vi "Read Image.vi"(0 "video in":refnum<class "MSC Video.lvclass">, 1 "image in":refnum<class "MSC Image.lvclass">, 5 "error in (no error)":errorcluster) -> (14 "video out":refnum<class "MSC Video.lvclass">, 15 "image out":refnum<class "MSC Image.lvclass">, 19 "error out":errorcluster)   [LabVIEW 2014, in "MSC Video.lvclass"]
doc: "Reads a frame from the camera and returns it as MSC Image.\nYou can use the image in connector to get around allocating and deallocation memory for each grabbed frame."
uses:
  MSC Video.lvclass
  MSC Image_class/MSC Image.lvclass
  MSC Video.lvclass/MSC Video.ctl
  Dependencies/x86/MSC I Process32.dll
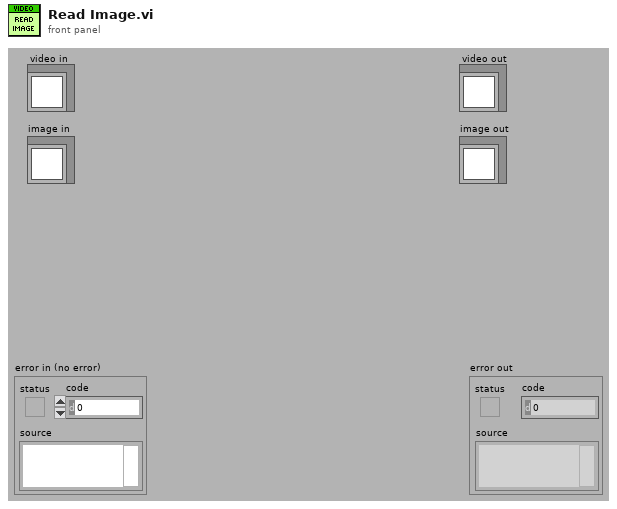
[diagram p1: front panel]
types:
  T1 = typedef "MSC Image.lvclass/Image.ctl" = cluster{"Pointer":u64, "Size":T2, "Image Type":T3, "Time Stamp":timestamp, "Variant":variant}
  T2 = typedef "MSC Image.lvclass/Size.ctl" = cluster{"Cols":i32, "Rows":i32}
  T3 = typedef "MSC Image.lvclass/Image Type.ctl" = i32
  T4 = typedef "MSC Video.lvclass/Video.ctl" = cluster{"Pointer":u64, "CamID":i32, "File Path":path, "Network Address":string, "opened":bool}
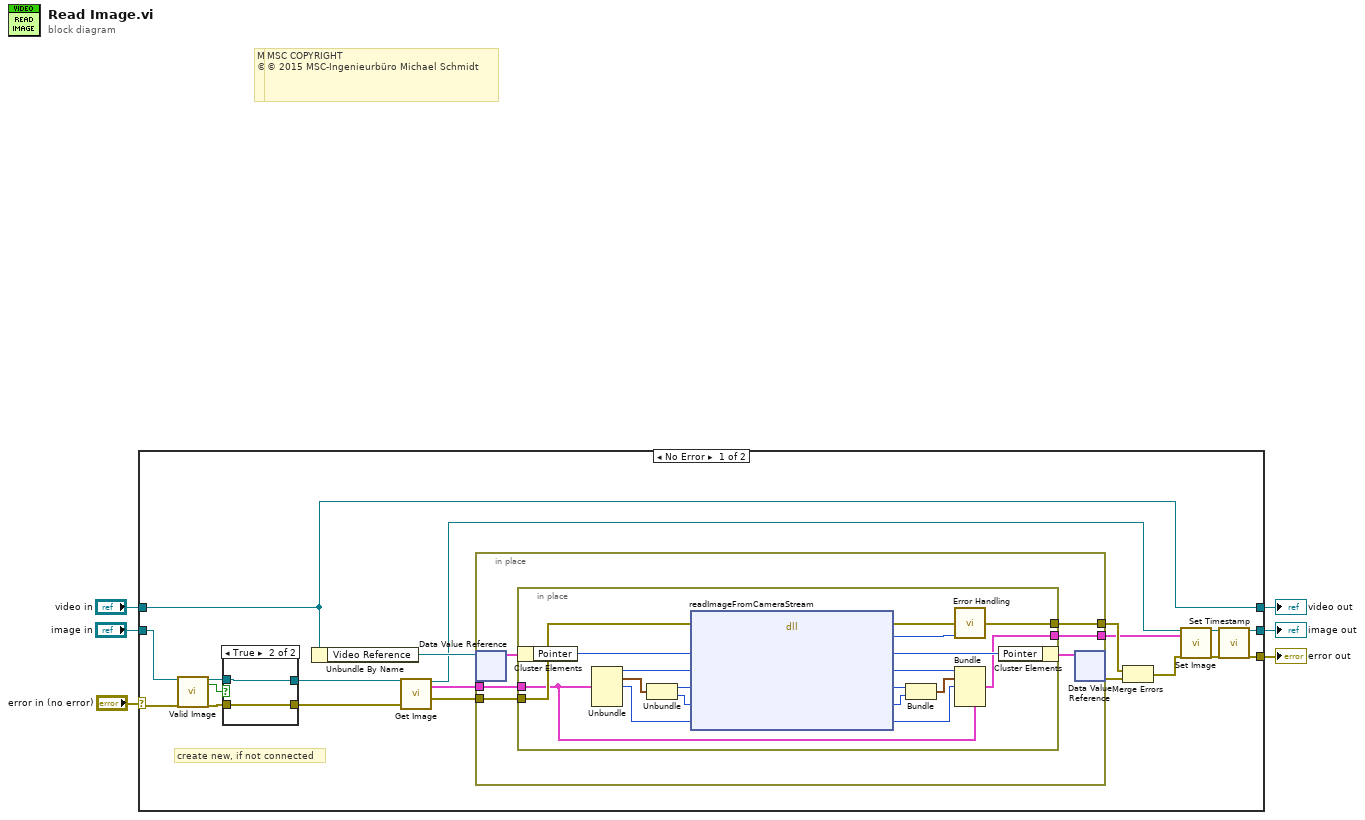
[diagram p0: block diagram]
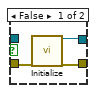
[diagram p2: hidden frame]
diagram:
  # "MSC COPYRIGHT\n© 2016 MSC-Ingenieurbüro Michael Schmidt"
  # "MSC COPYRIGHT\n© 2016 MSC-Ingenieurbüro Michael Schmidt"
  # "MSC COPYRIGHT\n© 2015 MSC-Ingenieurbüro Michael Schmidt"
  n1 = case shown="No Error" "error in (no error)" {
    selector: "error in (no error)" -> [w12 w58]
    tunnel: [w15 w58] -> w3
    tunnel: "video in" -> [w20 w57]
    tunnel: [w20 w57] -> w4
    tunnel: [w16 w56] -> w2
    tunnel: "image in" -> [w13 w56]
    frame No Error {
      # "create new, if not connected"
      n2 = call-dynamic "Valid Image.vi"("image in"=w13, "error in (no error)"=w12) -> ("image out"=w8:refnum<class "MSC Image.lvclass">, "Valid Image?"=w11:bool, "error out"=w9:errorcluster)  [unwired: 15 in]
      n3 = case shown="True" w11 {
        tunnel: [w28 w31] -> w10
        tunnel: w9 -> [w27 w31]
        tunnel: w8 -> [_ w30]
        tunnel: [w29 w30] -> w7
        frame False {
          n4 = call "Initialize.vi"("error in (no error)"=w27) -> ("image out"=w29:refnum<class "MSC Image.lvclass">, "error out"=w28:errorcluster)  [unwired: 17 in]
        }
        frame True {
        }
      }
      n5 = Unbundle By Name(w20) -> ("Video Reference"=w21:refnum<data-value>)
      n6 = call-dynamic "Get Image.vi"("image in"=w7, "error in (no error)"=w10) -> ("image out"=w18:refnum<class "MSC Image.lvclass">, "Image"=w24:T1, "error out"=w23:errorcluster)  [unwired: 15 in]
      n7 = in-place {
        in-place-border: w23 -> [w35]
        in-place-border: [w34] -> w25
        in-place-border: w24 -> [w33]
        in-place-border: [w32] -> w19
        n8 = in-place-dvr #1(w21) -> (w36:T4)  [unwired: 1 out]
        n9 = in-place {
          in-place-border: w35 -> [w39]
          in-place-border: [w42] -> w34
          in-place-border: w33 -> [w38]
          in-place-border: [w40] -> w32
          n10 = in-place-cluster #2(w36) -> ("Pointer"=w43:u64)
          n11 = Unbundle(w38) -> ("Pointer"=w44:u64, "Size"=w48:T2, "Image Type"=w47:T3)  [unwired: 2 out]
          n12 = Unbundle(w48) -> ("Cols"=w45:i32, "Rows"=w46:i32)
          n13 = dll-call lib="C:/Users/MSC/LabVIEW Projekte/LV 2014/MSC I-Process/user.lib/MSC-I Process/Dependencies/x86/MSC I Process*.dll" fn="readImageFromCameraStream"(error in=w39, "streamPointer"=w43, "pointer"=w44, "cols"=w45, "rows"=w46, "type"=w47) -> (error out=w54:errorcluster, "error"=w55:i32, "streamPointer"=w41:u64, "pointer"=w52:u64, "cols"=w50:i32, "rows"=w51:i32, "type"=w53:i32)  [unwired: 2 in, 1 out]
          n14 = Bundle("cols"=w50, "rows"=w51) -> (w49:cluster{"cols":i32, "rows":i32})  [unwired: 1 in]
          n15 = call "Error Handling.vi"("error in (no error)"=w54, "return type"=w55) -> ("error out"=w42:errorcluster)  [unwired: 12 in, 1 out]
          n16 = Bundle(cluster=w38, "Pointer"=w52, "Size"=w49, "Image Type"=w53) -> (w40:T1)  [unwired: 2 in]
          n17 = in-place-cluster #2("Pointer"=w41) -> (w37:T4)
        }
        n18 = in-place-dvr #1(w37) -> (w26:errorcluster)  [unwired: 1 out]
      }
      n19 = Merge Errors(w25, w26) -> (w22:errorcluster)
      n20 = call-dynamic "Set Image.vi"("image in"=w18, "Image"=w19, "error in (no error)"=w22) -> ("image out"=w17:refnum<class "MSC Image.lvclass">, "error out"=w14:errorcluster)  [unwired: 15 in]
      n21 = call-dynamic "Set Timestamp.vi"("image in"=w17, "error in (no error)"=w14) -> ("image out"=w16:refnum<class "MSC Image.lvclass">, "error out"=w15:errorcluster)  [unwired: 16 in]
    }
    frame Error {
    }
  }
  "error out" <- w3
  "video out" <- w4
  "image out" <- w2
